vi "Register for Waveform Data Events.vi"   [LabVIEW 2020, in "NI_VS Waveform Streaming Interface.lvlib"]
doc: "Registers to receive waveform data from the specified <B>WaveformStreamSpecifications</B>. You can use this VI prior to starting waveform streams to generate an event registration refnum that allows an Event structure to stream data from waveforms. You must manually select the instance to use."
uses:
  <vilib>/NI VeriStand/Execution/WaveformStreaming/NI_VS Waveform Streaming Interface.lvlib
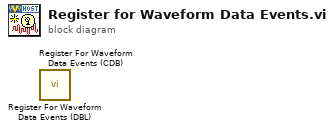
[diagram p0: block diagram]
diagram:
  n1 = call <vilib>:"Register For Waveform Data Events (DBL).vi"() -> ()  [unwired: 8 in, 4 out]
  n2 = call <vilib>:"Register For Waveform Data Events (CDB).vi"() -> ()  [unwired: 8 in, 4 out]
